vi "Step Start Action.vi"(8 "error in (no error)":errorcluster, 10 "Step in":refnum<class "Step.lvclass">, 11 "Tester in":refnum<class "Tester.lvclass">) -> (0 "error out":errorcluster, 2 "Step out":refnum<class "Step.lvclass">, 3 "Tester out":refnum<class "Tester.lvclass">)   [LabVIEW 2020, in "Tester.lvlib" / "Tester.lvclass"]
uses:
  Tester.lvclass
  Step/Step.lvclass
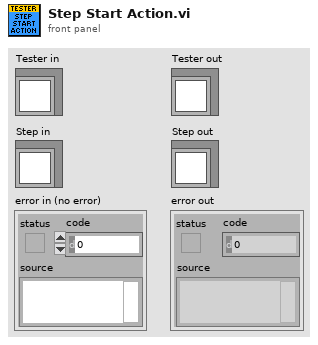
[diagram p1: front panel]
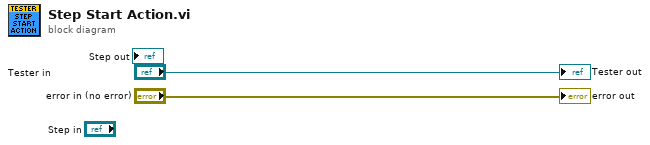
[diagram p0: block diagram]
diagram:
  "error out" <- "error in (no error)"
  "Tester out" <- "Tester in"
